vi "AutoCrossCourt.vi"(8 "error in (no error)":errorcluster, 10 "Starting Side":enum16{"Left", "Right", ""}(ring), 11 "Hot?":bool) -> (0 "error out":errorcluster)   [LabVIEW 2013]
uses:
  AutoWaitForHotStates.ctl
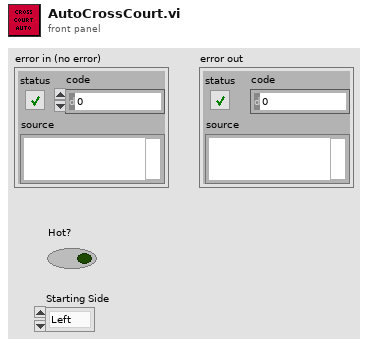
[diagram p1: front panel]
types:
  T1 = typedef "AutoWaitForHotStates.ctl" = enum16{"Check Hot", "Delay", "Fire", "Done"}
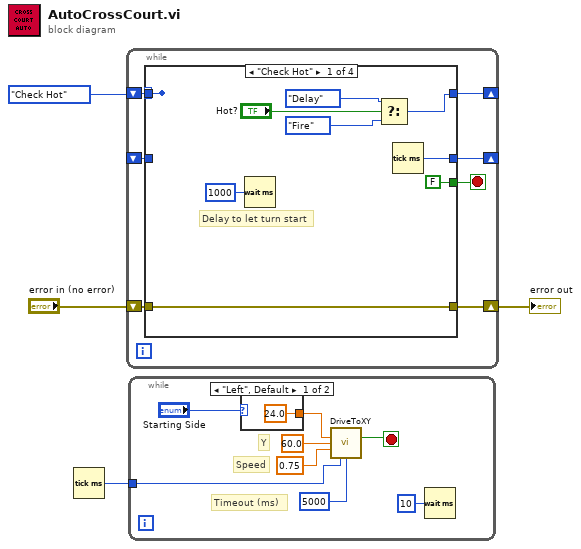
[diagram p0: block diagram]
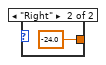
[diagram p2: hidden frame]
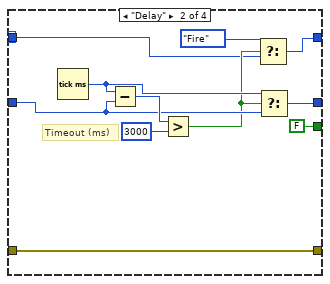
[diagram p3: hidden frame]
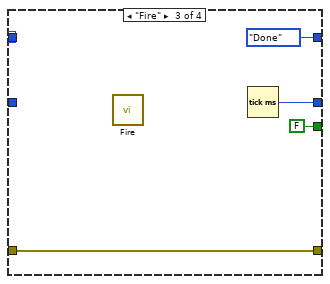
[diagram p4: hidden frame]
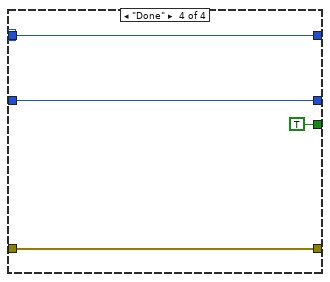
[diagram p5: hidden frame]
diagram:
  n1 = Tick Count (ms)() -> (millisecond timer value=w1:u32)
  n2 = while {
    shift-right: [w10] -> w4
    shift-left: "error in (no error)" -> [w11]
    shift-right: [w8] -> _
    shift-left: _ -> [w9]
    shift-right: [w5] -> _
    shift-left: AutoWaitForHotStates."Check Hot" -> [w6]
    stop <- w7 stop-if-true
    n3 = case shown="\"Check Hot\"" w6 {
      selector: w6 -> [_ w24 _ w36]
      tunnel: w11 -> [w15 w22 w34 w35]
      tunnel: [w15 w22 w34 w35] -> w10
      tunnel: [w18 w23 AutoWaitForHotStates."Done" w36] -> w5
      tunnel: w9 -> [_ w27 _ w37]
      tunnel: [w17 w25 w32 w37] -> w8
      tunnel: [FALSE FALSE FALSE TRUE] -> w7
      tunnel: w6 -> [_ _ _ _]
      frame "Check Hot" {
        # "Delay to let turn start"
        n4 = Wait (ms)(milliseconds to wait=u32 1000) -> ()  [unwired: 1 out]
        n5 = Select(t=AutoWaitForHotStates."Delay", s="Hot?", f=AutoWaitForHotStates."Fire") -> (s? t:f=w18:T1)
        n6 = Tick Count (ms)() -> (millisecond timer value=w17:u32)
      }
      frame "Delay" {
        # "Timeout (ms)"
        n7 = Tick Count (ms)() -> (millisecond timer value=w30:u32)
        n8 = Subtract(x=w30, y=w27) -> (x-y=w29:u32)
        n9 = Greater?(x=w29, y=u32 3000) -> (0:w26:bool)
        n10 = Select(t=AutoWaitForHotStates."Fire", s=w26, f=w24) -> (s? t:f=w23:T1)
        n11 = Select(t=w30, s=w26, f=w27) -> (s? t:f=w25:u32)
      }
      frame "Fire" {
        n12 = call "Fire.vi"() -> ()  [unwired: 11 in, 1 out]
        n13 = Tick Count (ms)() -> (millisecond timer value=w32:u32)
      }
      frame "Done" {
      }
    }
  }
  "error out" <- w4
  n14 = while {
    tunnel: w1 -> [w42]
    stop <- w43 stop-if-true
    # "Timeout (ms)"
    # "Speed"
    # "Y"
    n15 = case shown="\"Left\", Default" "Starting Side" {
      tunnel: [24.0 ("X Target") -24.0 ("X Target")] -> w39
      frame "Left", Default {
      }
      frame "Right" {
      }
    }
    n16 = call "DriveToXY.vi"("X Target"=w39, "Y Target"=60.0, "Speed"=0.75, "Start time"=w42, "Timeout (ms)"=u32 5000 ("y")) -> ("At Target"=w43:bool)  [unwired: 7 in, 3 out]
    n17 = Wait (ms)(milliseconds to wait=u32 10) -> ()  [unwired: 1 out]
  }
